vi "KB-内环象限选择.vi"(11 "象限选择":dbl[](array[numeric])) -> (2 "内环高度差":dbl, 3 "内环最高点":dbl)   [LabVIEW 2015]
panel:
  out "数组 4":dbl[](array[numeric])
  out "数组 3":string[](array[string])
  out "数组":i32[](array[numeric])
  # "Top\nBottom\nLeft\nRight"
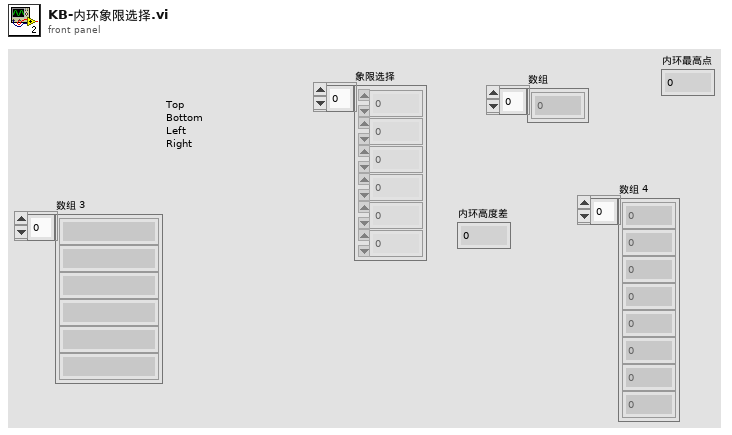
[diagram p1: front panel]
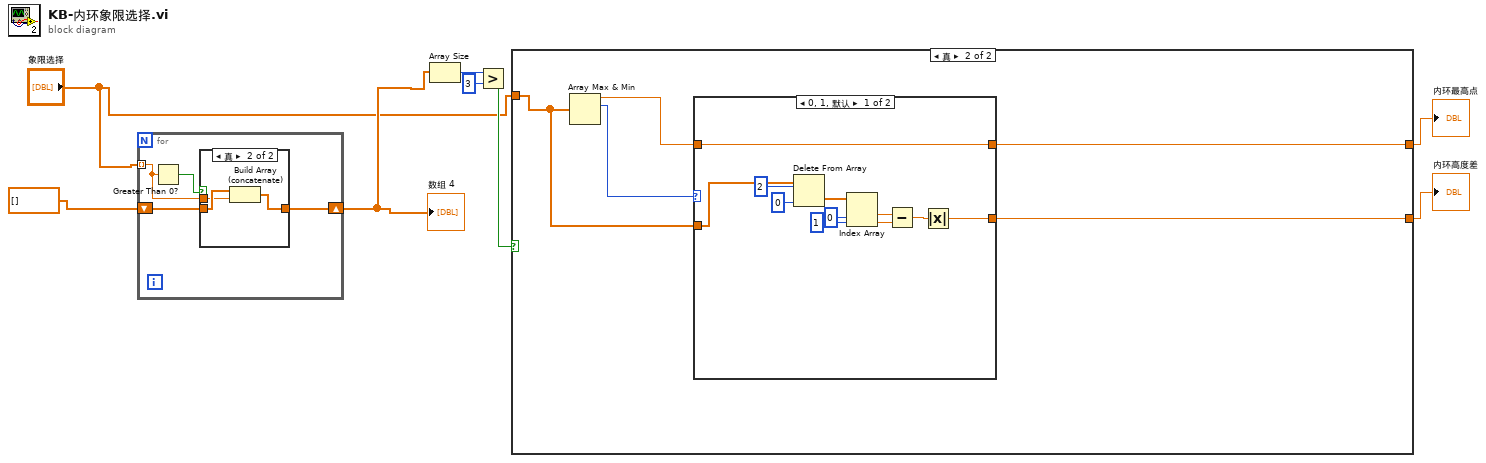
[diagram p0: block diagram]
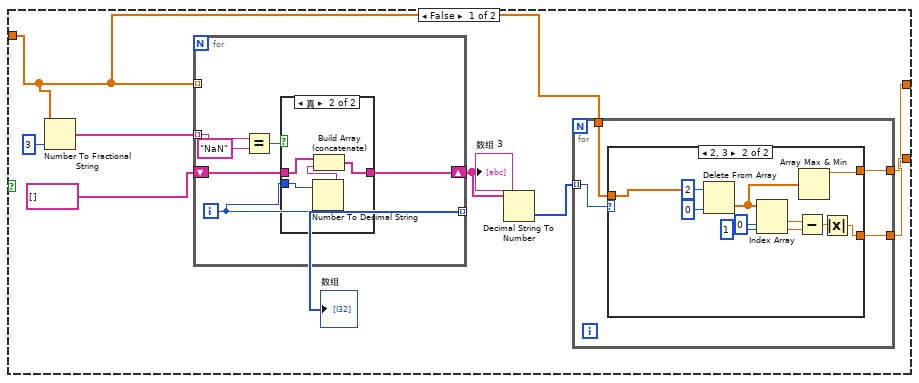
[diagram p3: hidden frame]
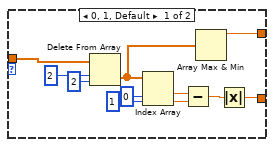
[diagram p4: hidden frame]
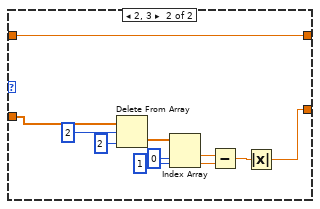
[diagram p6: hidden frame]
diagram:
  n1 = for {
    shift-right: [w10] -> w2
    shift-left: dbl[] [] -> [w11]
    tunnel: "象限选择" -> [w9] mode=indexing
    n2 = Greater Than 0?(x=w9) -> (x > 0?=w12:bool)
    n3 = case shown="真" w12 {
      tunnel: w11 -> [w13 w16]
      tunnel: [w13 w15] -> w10
      tunnel: w9 -> [_ w14]
      frame False {
      }
      frame True {
        n4 = Build Array (concatenate)(w16, w14) -> (w15:dbl[])
      }
    }
  }
  "数组 4" <- w2
  n5 = Array Size(array=w2) -> (size(s)=w8:i32)
  n6 = Greater?(x=w8, y=3) -> (0:w6:bool)
  n7 = case shown="真" w6 {
    tunnel: "象限选择" -> [w19 w63]
    tunnel: [w18 w65] -> w5
    tunnel: [w17 w64] -> w4
    frame False {
      n8 = Number To Fractional String(number=w19, precision (6)=i16 3 ("精度(6)")) -> (F-format string=w23:string[])  [unwired: 2 in]
      n9 = for {
        tunnel: w19 -> [_] mode=indexing
        tunnel: [w52] -> w25 mode=indexing
        tunnel: w23 -> [w57] mode=indexing
        shift-right: [w53] -> w21
        shift-left: string[] [] -> [w54]
        i -> [w52]
        n10 = Equal?(x=w57, y="NaN") -> (x = y?=w55:bool)
        n11 = case shown="真" w55 {
          tunnel: w54 -> [w58 w62]
          tunnel: [w58 w61] -> w53
          tunnel: w52 -> [_ w60]
          frame False {
          }
          frame True {
            n12 = Number To Decimal String(number=w60) -> (decimal integer string=w59:string)  [unwired: 1 in]
            n13 = Build Array (concatenate)(w62, w59) -> (w61:string[])
          }
        }
      }
      "数组" <- w25
      "数组 3" <- w21
      n14 = Decimal String To Number(string=w21) -> (number=w20:i32[])  [unwired: 2 in, 1 out]
      n15 = for {
        tunnel: w20 -> [w29] mode=indexing
        tunnel: w19 -> [w28]
        tunnel: [w27] -> w18
        tunnel: [w26] -> w17
        n16 = case shown="2, 3" w29 {
          tunnel: w28 -> [w33 w44]
          tunnel: [w32 w43] -> w27
          tunnel: [w30 w41] -> w26
          frame 0, 1, Default {
            n17 = Delete From Array(array=w33, length=2 ("长度"), index=2 ("索引")) -> (deleted portion=w31:dbl[])  [unwired: 1 out]
            n18 = Index Array(array=w31, index #1=0 ("索引"), index #2=1 ("索引")) -> (element #1=w36:dbl, element #2=w35:dbl)
            n19 = Subtract(x=w36, y=w35) -> (x-y=w34:dbl)
            n20 = Array Max & Min(array=w31) -> (max value=w30:dbl)  [unwired: 3 out]
            n21 = Absolute Value(x=w34) -> (abs(x)=w32:dbl)
          }
          frame 2, 3 {
            n22 = Delete From Array(array=w44, length=2 ("长度"), index=0 ("索引")) -> (deleted portion=w42:dbl[])  [unwired: 1 out]
            n23 = Index Array(array=w42, index #1=0 ("索引"), index #2=1 ("索引")) -> (element #1=w47:dbl, element #2=w46:dbl)
            n24 = Subtract(x=w47, y=w46) -> (x-y=w45:dbl)
            n25 = Array Max & Min(array=w42) -> (max value=w41:dbl)  [unwired: 3 out]
            n26 = Absolute Value(x=w45) -> (abs(x)=w43:dbl)
          }
        }
      }
    }
    frame True {
      n27 = Array Max & Min(array=w63) -> (max value=w66:dbl, max index (indices)=w67:i32)  [unwired: 2 out]
      n28 = case shown="0, 1, 默认" w67 {
        tunnel: w63 -> [w78 w81]
        tunnel: w66 -> [w68 w79]
        tunnel: [w70 w80] -> w65
        tunnel: [w68 w79] -> w64
        frame 0, 1, Default {
          n29 = Delete From Array(array=w78, length=2 ("长度"), index=0 ("索引")) -> (deleted portion=w69:dbl[])  [unwired: 1 out]
          n30 = Index Array(array=w69, index #1=0 ("索引"), index #2=1 ("索引")) -> (element #1=w73:dbl, element #2=w72:dbl)
          n31 = Subtract(x=w73, y=w72) -> (x-y=w71:dbl)
          n32 = Absolute Value(x=w71) -> (abs(x)=w70:dbl)
        }
        frame 2, 3 {
          n33 = Delete From Array(array=w81, length=2 ("长度"), index=2 ("索引")) -> (deleted portion=w87:dbl[])  [unwired: 1 out]
          n34 = Index Array(array=w87, index #1=0 ("索引"), index #2=1 ("索引")) -> (element #1=w84:dbl, element #2=w83:dbl)
          n35 = Subtract(x=w84, y=w83) -> (x-y=w82:dbl)
          n36 = Absolute Value(x=w82) -> (abs(x)=w80:dbl)
        }
      }
    }
  }
  "内环高度差" <- w5
  "内环最高点" <- w4
